vi "Create AO Tasks.vi"(8 "error in (no error)":errorcluster, 11 "DAQmx in":refnum<class "DAQmx.lvclass">) -> (0 "error out":errorcluster, 3 "DAQmx out":refnum<class "DAQmx.lvclass">)   [LabVIEW 2019, in "DAQmx.lvclass"]
uses:
  DAQmx.lvclass
  DAQmx.lvclass/DAQmx.ctl
  <vilib>/DAQmx/create/channels.llb/DAQmx Create Channel (AO-Voltage-Basic).vi
  <resource>/objmgr/daqmx.rc
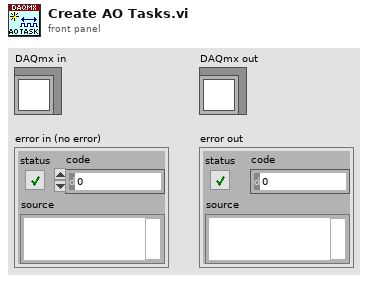
[diagram p1: front panel]
types:
  T1 = typedef "DAQmx.lvclass/DAQ.Config.AO--Cluster--Array.ctl" = T2[]
  T2 = typedef "DAQmx.lvclass/DAQ.Config.AO--Cluster.ctl" = cluster{"Channels":tag, "Range":T3, "output terminal configuration":i32, "Type":T4}
  T3 = typedef "DAQmx.lvclass/DAQ.Config.AO.Range--enum.ctl" = enum16{"±0.1", "±1.0", "±10.0", ""}
  T4 = typedef "DAQmx.lvclass/DAQ.Config.Device Type--enum.ctl" = enum16{"None", "USB-4431", "PXI-446x"}
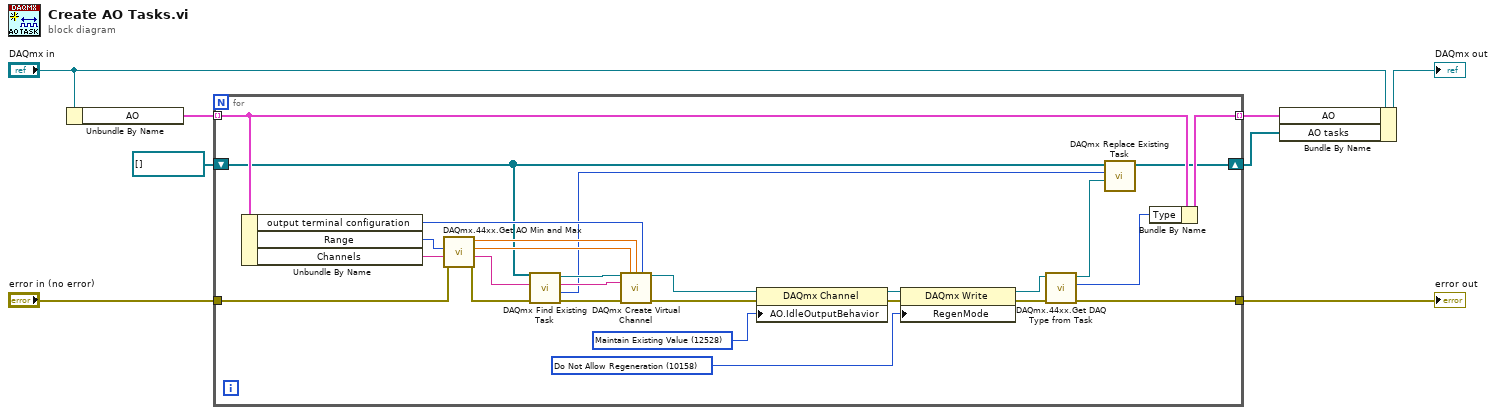
[diagram p0: block diagram]
diagram:
  n1 = Unbundle By Name("DAQmx in") -> ("AO"=w3:T1)
  n2 = for {
    tunnel: "error in (no error)" -> [w29]
    tunnel: [w21] -> w1
    tunnel: w3 -> [w30] mode=indexing
    tunnel: [w31] -> w4 mode=indexing
    shift-right: [w13] -> w5
    shift-left: refnum<k21>[] [] -> [w10]
    w17 = 10158 items=["Allow Regeneration"=10097, "Do Not Allow Regeneration"=10158] ("RegenMode")
    w16 = 12528 items=["Zero Volts"=12526, "High-Impedance"=12527, "Maintain Existing Value"=12528] ("AO.IdleOutputBehavior")
    n3 = Unbundle By Name(w30) -> ("output terminal configuration"=w32:i32, "Range"=w28:T3, "Channels"=w33:tag)
    n4 = call "DAQmx.44xx.Get AO Min and Max.vi"("error in (no error)"=w29, "AO.channels"=w33, "AO.Range"=w28) -> ("error out"=w25:errorcluster, "AO.channels out"=w27:tag, "AO.max"=w35:dbl, "AO.min"=w34:dbl)  [unwired: 5 in]
    n5 = call "DAQmx Find Existing Task.vi"("error in (no error)"=w25, "Channels"=w27, "Tasks in"=w10) -> ("error out"=w24:errorcluster, "Task Index"=w11:i32, "Channel out"=w26:tag, "Task out"=w23:refnum<k21>)  [unwired: 5 in]
    n6 = call-poly <vilib>:"DAQmx Create Virtual Channel.vi"("task in"=w23, "maximum value"=w35, "minimum value"=w34, "output terminal configuration"=w32, "physical channels"=w26, "error in"=w24) -> ("task out"=w15:refnum<k21>, "error out"=w20:errorcluster)  [unwired: 8 in]
    n7 = property class="DAQmx Channel"(reference=w15, error in=w20, "AO.IdleOutputBehavior"=w16) -> (reference out=w19:refnum<k21>, error out=w18:errorcluster)
    n8 = property class="DAQmx Write"(reference=w19, error in=w18, "RegenMode"=w17) -> (reference out=w14:refnum<k21>, error out=w22:errorcluster)
    n9 = call "DAQmx.44xx.Get DAQ Type from Task.vi"("error in (no error)"=w22, "Task in"=w14) -> ("error out"=w21:errorcluster, "DAQ Type"=w9:T4, "Task out"=w12:refnum<k21>)  [unwired: 6 in, 1 out]
    n10 = call "DAQmx Replace Existing Task.vi"("Task in"=w12, "Task Index"=w11, "Tasks in"=w10) -> ("Tasks out"=w13:refnum<k21>[])  [unwired: 8 in]
    n11 = Bundle By Name(cluster=w30, "Type"=w9) -> (w31:T2)
  }
  "error out" <- w1
  n12 = Bundle By Name(cluster="DAQmx in", "AO"=w4, "AO tasks"=w5) -> (→"DAQmx out":refnum<class "DAQmx.lvclass">)
